vi "Write Slow FPGA Telem to TDMS.vi"   [LabVIEW 2015]
uses:
  FPGA Telem for Slow Logging.ctl
  Global Data.vi
types:
  T1 = enum16{"open", "open or create", "create or replace", "create", "open (read-only)"}
  T2 = cluster{"read mode":enum16{"polling", "blocking"}, "write mode":enum16{"polling", "blocking"}}
  T3 = typedef "FPGA Telem for Slow Logging.ctl" = cluster{"TSBRIO":fxp<+/-,16,9>, "VsbRIOSpply":fxp<+/-,25,6>, "bFPGALED":bool, "CPU Load":cluster{"Total (%)":dbl, "Time Critical (%)":dbl, "Timed Structures (%)":dbl, "High (%)":dbl, "Above Normal (%)":dbl, "Normal (%)":dbl, "Background (%)":dbl, "Idle (%)":dbl, "ISR (%)":dbl}, "Time Stamp":timestamp, "NLatiPhone":dbl, "NLongiPhone":dbl, "nGPSiPhone":dbl, "IHighCurrent":fxp<+/-,24,15>, "ILowCurrent":fxp<+/-,24,15>, "V5VSupply":fxp<+/-,24,5>, "tCurrentLap":u32, "tLastLap":u32, "NLap":u8, "bCoolantPumpEnable":bool, "bRTDSEnable":bool, "bTSMSInStatus":bool, "bPosAIREnable":bool, "bBMSOK":bool, "bIMDOK":bool, "bBSPDOK":bool, "bSBRIOOK2":bool, "bSBRIOOK1":bool, "bTSMSOutStatus":bool, "bMotorControllerEnable":bool, "Tire Diameter(m)":fxp<+,16,1>}
  T4 = cluster{"Total (%)":dbl, "Time Critical (%)":dbl, "Timed Structures (%)":dbl, "High (%)":dbl, "Above Normal (%)":dbl, "Normal (%)":dbl, "Background (%)":dbl, "Idle (%)":dbl, "ISR (%)":dbl}
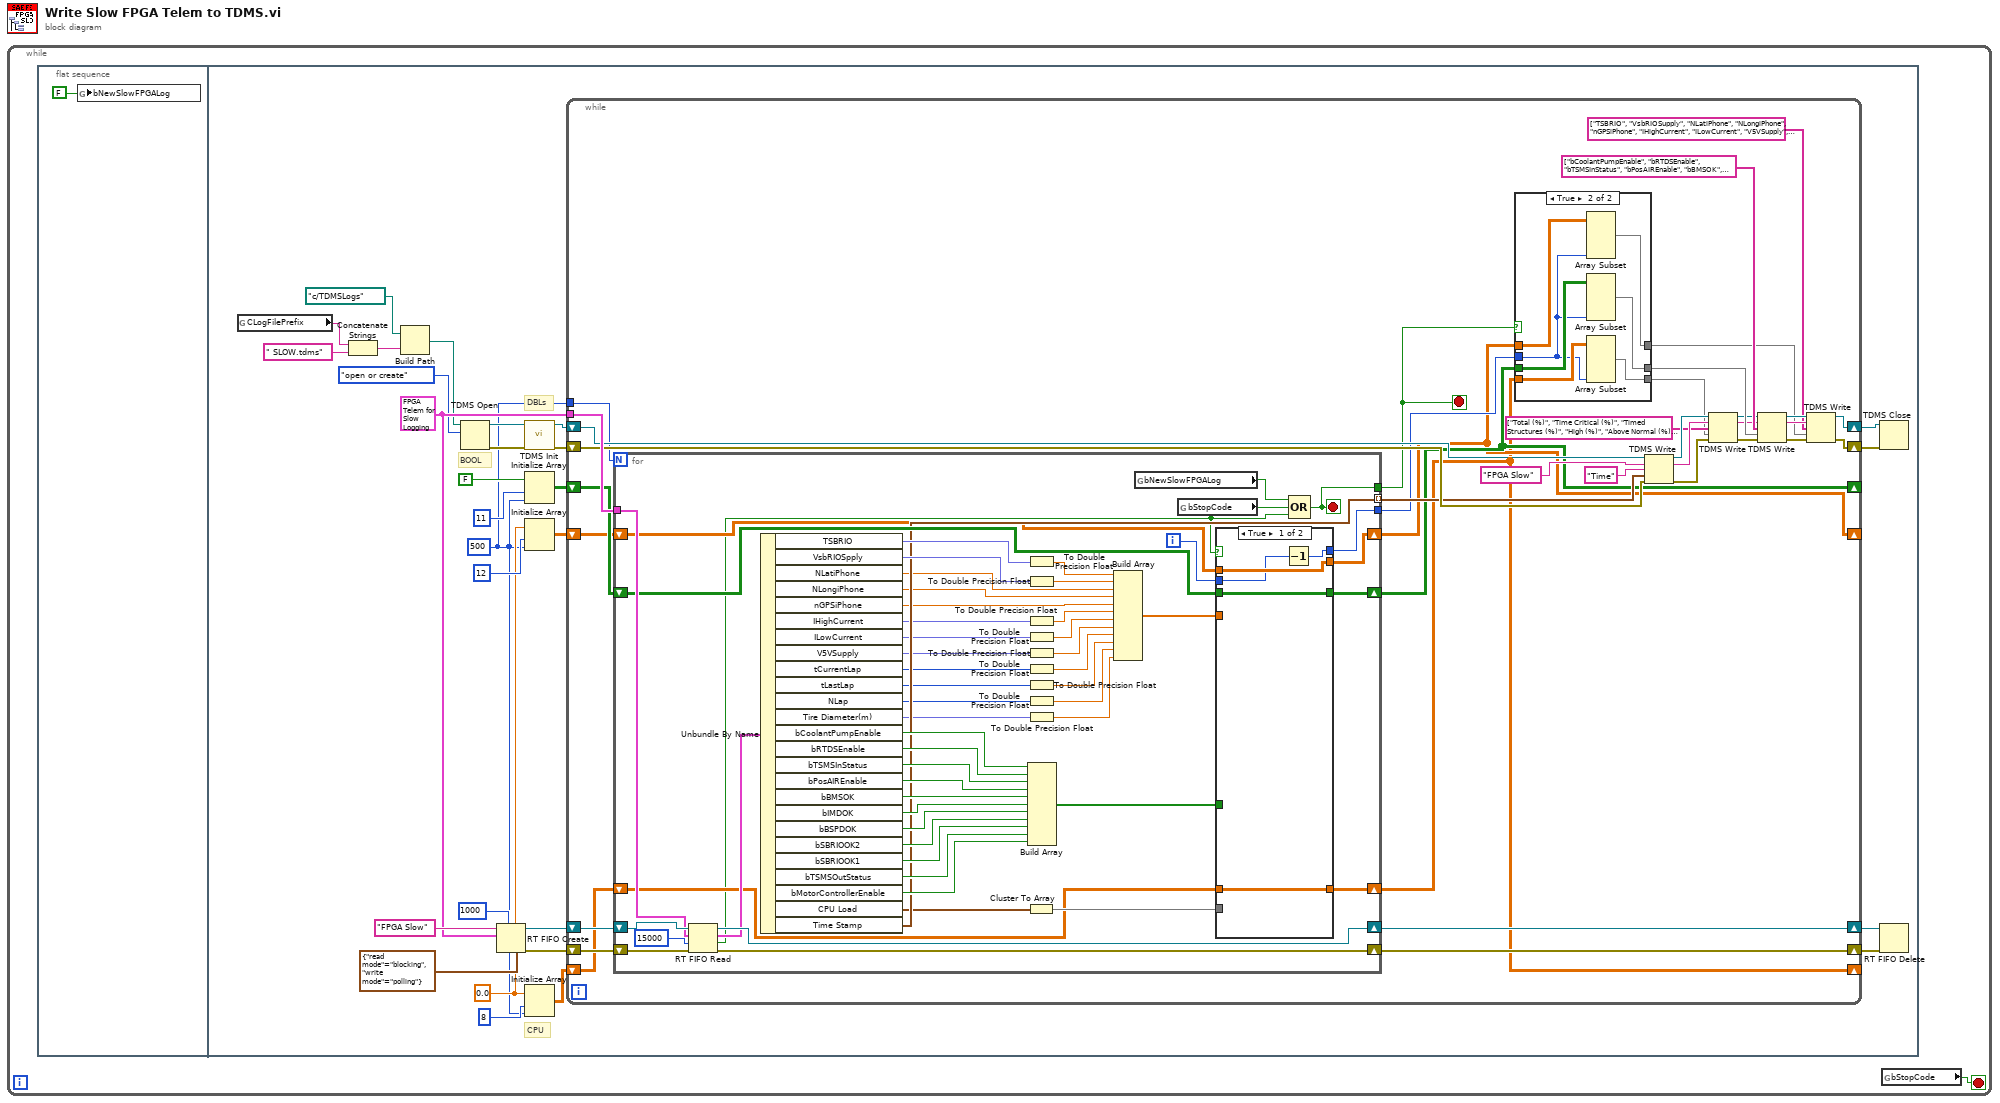
[diagram p0: block diagram]
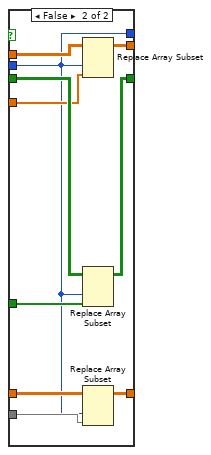
[diagram p3: hidden frame]
diagram:
  n1 = while {
    stop <- w1 stop-if-true
    n2 = flat-sequence {
      frame #0 {
        n3 = global write "Global Data.vi" "bNewSlowFPGALog"(FALSE ("New S_FPGA TDMS")) -> ()
      }
      frame #1 {
        w9 = 0.0 ("Total (%)")
        w6 = 500 ("dimension size")
        w26 = T3 {"TSBRIO"=0.0, "VsbRIOSpply"=0.0, "bFPGALED"=FALSE, "CPU Load"={"Total (%)"=0.0, "Time Critical (%)"=0.0, "Timed Structures (%)"=0.0, "High (%)"=0.0, "Above Normal (%)"=0.0, "Normal (%)"=0.0, "Background (%)"=0.0, "Idle (%)"=0.0, "ISR (%)"=0.0}, "Time Stamp"=timestamp(0 s since 1904-01-01), "NLatiPhone"=0.0, "NLongiPhone"=0.0, "nGPSiPhone"=0.0, "IHighCurrent"=0.0, "ILowCurrent"=0.0, "V5VSupply"=-16.0, "tCurrentLap"=4, "tLastLap"=0, "NLap"=0, "bCoolantPumpEnable"=FALSE, "bRTDSEnable"=FALSE, "bTSMSInStatus"=FALSE, "bPosAIREnable"=FALSE, "bBMSOK"=TRUE, "bIMDOK"=TRUE, "bBSPDOK"=FALSE, "bSBRIOOK2"=FALSE, "bSBRIOOK1"=FALSE, "bTSMSOutStatus"=FALSE, "bMotorControllerEnable"=FALSE, "Tire Diameter(m)"=0.0} ("FPGA Logging Telem")
        # "CPU"
        # "BOOL"
        # "DBLs"
        n4 = global read "Global Data.vi" "CLogFilePrefix"() -> (w5:string)
        n5 = Concatenate Strings(w5, " SLOW.tdms" ("string")) -> (w3:string)
        n6 = Build Path(base path=path "c:/TDMSLogs", name or relative path=w3) -> (appended path=w25:path)
        n7 = TDMS Open(10:T1."open or create" ("operation (0:open)"), 11:w25) -> (0:w19:errorcluster, 3:w20:refnum<k34>)  [unwired: 5 in]
        n8 = RT FIFO Create(0:"FPGA Slow" ("name (unnamed)"), 1:w26, 4:u32 1000 ("size (10)"), 7:T2 {"read mode"=enum."blocking", "write mode"=enum."polling"} ("r/w modes (polling,polling)")) -> (8:w28:refnum<k33>, 11:w27:errorcluster)  [unwired: 4 in, 1 out]
        n9 = call "TDMS Init.vi"("error in (no error)"=w19, "tdms file"=w20) -> ("error out"=w17:errorcluster, "tdms file out"=w18:refnum<k34>)  [unwired: 8 in]
        n10 = Initialize Array(FALSE ("Brake Light Out"), 11 ("dimension size"), w6) -> (w11:bool[][])
        n11 = Initialize Array(w9, 12 ("dimension size"), w6) -> (w10:dbl[][])
        n12 = Initialize Array(w9, 8 ("dimension size"), w6) -> (w7:dbl[][])
        n13 = while {
          tunnel: w26 -> [w65]
          shift-right: [w64] -> w15
          shift-left: w28 -> [w67]
          shift-right: [w63] -> w16
          shift-left: w27 -> [w66]
          shift-right: [w50] -> w22
          shift-left: w18 -> [w62]
          shift-right: [w49] -> w21
          shift-left: w17 -> [w61]
          shift-right: [w39] -> _
          shift-left: w11 -> [w48]
          shift-right: [w38] -> _
          shift-left: w10 -> [w45]
          shift-right: [w37] -> _
          shift-left: w7 -> [w44]
          tunnel: w6 -> [w36]
          stop <- w32 stop-if-true
          n14 = for {
            N: w36 -> [_]
            tunnel: w65 -> [w131]
            shift-right: [w129] -> w64
            shift-left: w67 -> [w133]
            shift-right: [w128] -> w63
            shift-left: w66 -> [w132]
            shift-right: [w109] -> w39
            shift-left: w48 -> [w111]
            tunnel: [w108] -> w47 mode=indexing
            shift-right: [w105] -> w38
            shift-left: w45 -> [w107]
            shift-right: [w101] -> w37
            shift-left: w44 -> [w102]
            tunnel: [w78] -> w43
            tunnel: [w80] -> w32
            i -> [w100]
            stop <- w80 stop-if-true
            n15 = RT FIFO Read(0:w133, 1:w131, 2:15000 ("timeout in ms (0)"), 3:w132) -> (8:w129:refnum<k33>, 9:w127:T3, 10:w79:bool, 11:w128:errorcluster)  [unwired: 1 out]
            n16 = Unbundle By Name(w127) -> ("TSBRIO"=w126:fxp<+/-,16,9>, "VsbRIOSpply"=w125:fxp<+/-,25,6>, "NLatiPhone"=w97:dbl, "NLongiPhone"=w96:dbl, "nGPSiPhone"=w95:dbl, "IHighCurrent"=w94:fxp<+/-,24,15>, "ILowCurrent"=w93:fxp<+/-,24,15>, "V5VSupply"=w90:fxp<+/-,24,5>, "tCurrentLap"=w88:u32, "tLastLap"=w87:u32, "NLap"=w86:u8, "Tire Diameter(m)"=w82:fxp<+,16,1>, "bCoolantPumpEnable"=w122:bool, "bRTDSEnable"=w121:bool, "bTSMSInStatus"=w120:bool, "bPosAIREnable"=w119:bool, "bBMSOK"=w118:bool, "bIMDOK"=w117:bool, "bBSPDOK"=w116:bool, "bSBRIOOK2"=w115:bool, "bSBRIOOK1"=w114:bool, "bTSMSOutStatus"=w113:bool, "bMotorControllerEnable"=w112:bool, "CPU Load"=w104:T4, "Time Stamp"=w108:timestamp)
            n17 = Cluster To Array(cluster=w104) -> (array=w103:dbl[])
            n18 = To Double Precision Float(number=w126) -> (double precision float=w124:dbl)
            n19 = To Double Precision Float(number=w125) -> (double precision float=w123:dbl)
            n20 = To Double Precision Float(number=w94) -> (double precision float=w92:dbl)
            n21 = To Double Precision Float(number=w93) -> (double precision float=w91:dbl)
            n22 = To Double Precision Float(number=w90) -> (double precision float=w89:dbl)
            n23 = To Double Precision Float(number=w88) -> (double precision float=w85:dbl)
            n24 = To Double Precision Float(number=w87) -> (double precision float=w84:dbl)
            n25 = To Double Precision Float(number=w86) -> (double precision float=w83:dbl)
            n26 = To Double Precision Float(number=w82) -> (double precision float=w81:dbl)
            n27 = Build Array(w122, w121, w120, w119, w118, w117, w116, w115, w114, w113, w112) -> (w110:bool[])
            n28 = Build Array(w124, w123, w97, w96, w95, w92, w91, w89, w85, w84, w83, w81) -> (w106:dbl[])
            n29 = global read "Global Data.vi" "bNewSlowFPGALog"() -> (w99:bool)
            n30 = global read "Global Data.vi" "bStopCode"() -> (w98:bool)
            n31 = case shown="True" w79 {
              tunnel: w111 -> [w138 w148]
              tunnel: w110 -> [_ w147]
              tunnel: [w138 w146] -> w109
              tunnel: w107 -> [w137 w145]
              tunnel: w106 -> [_ w144]
              tunnel: [w137 w143] -> w105
              tunnel: w103 -> [_ w142]
              tunnel: w102 -> [w136 w141]
              tunnel: [w136 w140] -> w101
              tunnel: w100 -> [w134 w139]
              tunnel: [w135 w139] -> w78
              frame True {
                n32 = Decrement(x=w134) -> (x-1=w135:i32)
              }
              frame False {
                n33 = Replace Array Subset(array=w145, new element=w144, index (col)=w139) -> (w143:dbl[][])  [unwired: 1 in]
                n34 = Replace Array Subset(array=w148, new element=w147, index (col)=w139) -> (w146:bool[][])  [unwired: 1 in]
                n35 = Replace Array Subset(array=w141, new element=w142, index (col)=w139) -> (w140:dbl[][])  [unwired: 1 in]
              }
            }
            n36 = Compound Arithmetic op=OR(w99, w98, w79) -> (w80:bool)
          }
          n37 = case shown="True" w32 {
            tunnel: w37 -> [w70 w77]
            tunnel: w39 -> [w69 w76]
            tunnel: w38 -> [w68 w75]
            tunnel: w43 -> [_ w74]
            tunnel: [w70 w73] -> w42
            tunnel: [w69 w72] -> w41
            tunnel: [w68 w71] -> w40
            frame False {
            }
            frame True {
              n38 = Array Subset(array=w75, length (col)=w74) -> (w71:dbl[][])  [unwired: 3 in]
              n39 = Array Subset(array=w76, length (col)=w74) -> (w72:bool[][])  [unwired: 3 in]
              n40 = Array Subset(array=w77, length (col)=w74) -> (w73:dbl[][])  [unwired: 3 in]
            }
          }
          n41 = TDMS Write(0:w62, 5:"FPGA Slow" ("group name in (Untitled)"), 7:"Time", 9:w47, 11:w61) -> (4:w59:refnum<k34>, 6:w57:string, 15:w58:errorcluster)  [unwired: 1 in, 1 out]
          n42 = TDMS Write(0:w59, 5:w57, 7:string[] ["Total (%)", "Time Critical (%)", "Timed Structures (%)", "High (%)", "Above Normal (%)", "Normal (%)", "Background (%)", "Idle (%)", "ISR (%)"] ("channel name(s) in (Untitled)"), 9:w42, 11:w58) -> (4:w35:refnum<k34>, 6:w34:string, 15:w33:errorcluster)  [unwired: 1 in, 1 out]
          n43 = TDMS Write(0:w35, 5:w34, 7:string[] ["bCoolantPumpEnable", "bRTDSEnable", "bTSMSInStatus", "bPosAIREnable", "bBMSOK", "bIMDOK", "bBSPDOK", "bSBRIOOK2", "bSBRIOOK1", "bTSMSOutStatus", "bMotorControllerEnable", "BSPD In", "Brake Light Out"] ("channel name(s) in (Untitled)"), 9:w41, 11:w33) -> (4:w54:refnum<k34>, 6:w52:string, 15:w53:errorcluster)  [unwired: 1 in, 1 out]
          n44 = TDMS Write(0:w54, 5:w52, 7:string[] ["TSBRIO", "VsbRIOSupply", "NLatiPhone", "NLongiPhone", "nGPSiPhone", "IHighCurrent", "ILowCurrent", "V5VSupply", "tCurrentLap", "tLastLap", "NLap", "Tire Diameter(m)"] ("channel name(s) in (Untitled)"), 9:w40, 11:w53) -> (4:w50:refnum<k34>, 15:w49:errorcluster)  [unwired: 1 in, 2 out]
        }
        n45 = TDMS Close(8:w21, 11:w22) -> ()  [unwired: 2 out]
        n46 = RT FIFO Delete(0:w15, 3:w16) -> ()  [unwired: 1 in, 1 out]
      }
    }
    n47 = global read "Global Data.vi" "bStopCode"() -> (w1:bool)
  }
